vi "SendTcpMessageBase.vi"(6 "timeout (5 sec)":i32=5000, 8 "error in (no error)":errorcluster, 10 "Message":T1, 11 "tcp in":refnum<k5>) -> (0 "error out":errorcluster, 1 "error57":bool, 3 "tcp out":refnum<k5>)   [LabVIEW 2017]
uses:
  <vilib>/addons/InsightCM/MessageBus/Base/controls/Message.ctl
  <vilib>/addons/InsightCM/MessageBus/Base/controls/MessageHeader.ctl
  <vilib>/addons/InsightCM/MessageBus/Base/controls/KeyValuePair.ctl
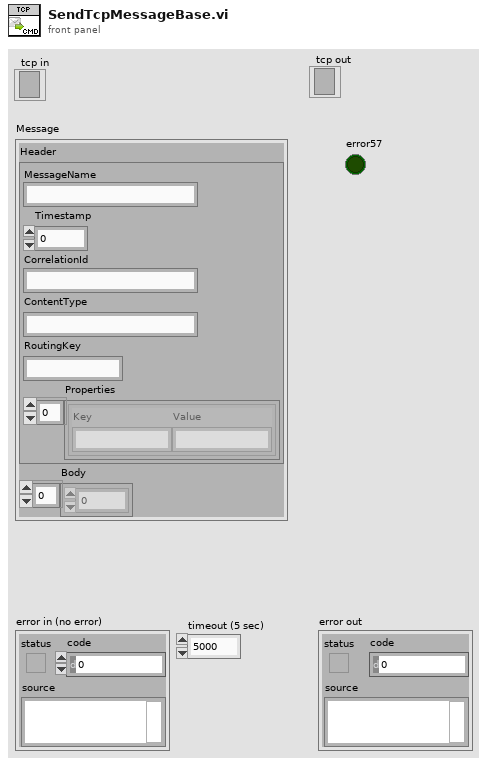
[diagram p1: front panel]
types:
  T1 = typedef "Message.ctl" = cluster{"Header":T2, "Body":u8[]}
  T2 = typedef "MessageHeader.ctl" = cluster{"MessageName":string, "Timestamp":i64, "CorrelationId":string, "ContentType":string, "RoutingKey":string, "Properties":T3[]}
  T3 = typedef "KeyValuePair.ctl" = cluster{"Key":string, "Value":string}
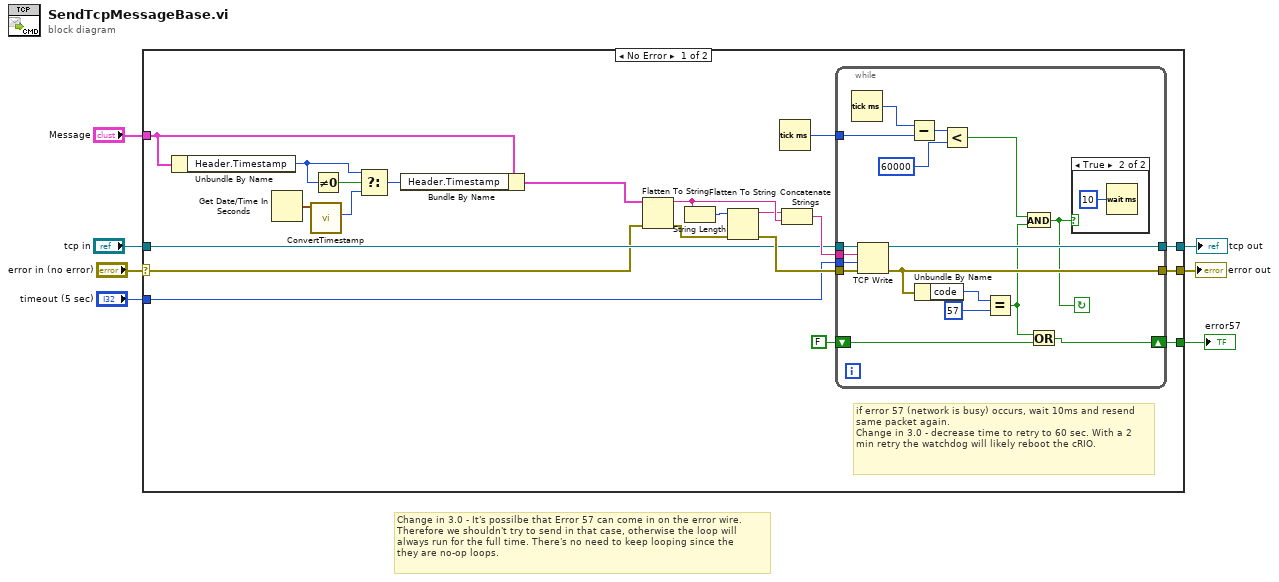
[diagram p0: block diagram]
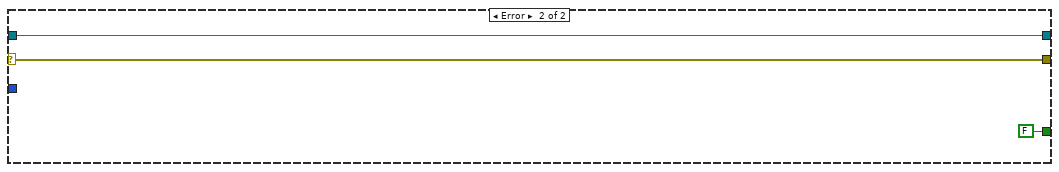
[diagram p3: hidden frame]
diagram:
  # "Change in 3.0 - It's possilbe that Error 57 can come in on the error wire.\nTherefore we shouldn't try to send in that case, otherwise the loop will \nalways run for the full time. There's no need to keep looping since the\nthey are no-op loops."
  n1 = case shown="No Error" "error in (no error)" {
    selector: "error in (no error)" -> [w8 w48]
    tunnel: [w28 w48] -> w7
    tunnel: "timeout (5 sec)" -> [w22 _]
    tunnel: "Message" -> [w15 _]
    tunnel: "tcp in" -> [w14 w49]
    tunnel: [w13 w49] -> w3
    tunnel: [w11 FALSE] -> w2
    frame No Error {
      # "if error 57 (network is busy) occurs, wait 10ms and resend same packet again.\nChange in 3.0 - decrease time to retry to 60 sec. With a 2 min retry the watchdog will likely reboot the cRIO."
      n2 = Unbundle By Name(w15) -> ("Header.Timestamp"=w19:i64)
      n3 = Get Date/Time In Seconds() -> (seconds since 1Jan1904=w18:timestamp)
      n4 = call <vilib>:"ConvertTimestamp.vi"("Time Stamp"=w18) -> ("Timestamp out"=w17:i64)  [unwired: 10 in]
      n5 = Not Equal To 0?(x=w19) -> (x != 0?=w20:bool)
      n6 = Select(t=w19, s=w20, f=w17) -> (s? t:f=w16:i64)
      n7 = Bundle By Name(cluster=w15, "Header.Timestamp"=w16) -> (w9:T1)
      n8 = Flatten To String(anything=w9, error in (no error)=w8) -> (data string=w24:string, error out=w26:errorcluster)  [unwired: 2 in, 1 out]
      n9 = String Length(string=w24) -> (length=w21:i32)
      n10 = Flatten To String(anything=w21, error in (no error)=w26) -> (data string=w23:string, error out=w27:errorcluster)  [unwired: 2 in, 1 out]
      n11 = Tick Count (ms)() -> (millisecond timer value=w12:u32)
      n12 = Concatenate Strings(w23, w24) -> (w25:string)
      n13 = while {
        tunnel: [w40] -> w28
        tunnel: w27 -> [w45]
        tunnel: w25 -> [w44]
        tunnel: w22 -> [w43]
        tunnel: w14 -> [w42]
        tunnel: [w41] -> w13
        tunnel: w12 -> [w36]
        shift-right: [w30] -> w11
        shift-left: FALSE -> [w29]
        stop <- w32 continue-if-true
        n14 = Tick Count (ms)() -> (millisecond timer value=w37:u32)
        n15 = TCP Write(connection ID=w42, data in=w44, error in (no error)=w45, 9:w43) -> (connection ID out=w41:refnum<k5>, error out=w40:errorcluster)  [unwired: 1 out]
        n16 = Subtract(x=w37, y=w36) -> (x-y=w35:u32)
        n17 = Unbundle By Name(w40) -> ("code"=w39:i32)
        n18 = Less?(x=w35, y=u32 60000) -> (x < y?=w33:bool)
        n19 = Equal?(x=w39, y=57) -> (x = y?=w31:bool)
        n20 = And(x=w33, y=w31) -> (x .and. y?=w32:bool)
        n21 = Or(x=w31, y=w29) -> (x .or. y?=w30:bool)
        n22 = case shown="True" w32 {
          frame False {
            # "no wait"
          }
          frame True {
            n23 = Wait (ms)(milliseconds to wait=u32 10) -> ()  [unwired: 1 out]
          }
        }
      }
    }
    frame Error {
    }
  }
  "error out" <- w7
  "tcp out" <- w3
  "error57" <- w2
